vi "look up indices.vi"(8 "error in":errorcluster, 9 "output dictionary":refnum<class "data dictionary.lvclass">, 10 "input dictionary":refnum<class "data dictionary.lvclass">, 11 "slave data subsets":T4[](array[typedef])) -> (0 "error out":errorcluster, 2 "outputs":T1[](array[typedef]), 3 "inputs":T1[](array[typedef]))   [LabVIEW 2013, in "Profibus Module runtime.lvclass"]
uses:
  Profibus Module runtime.lvclass
  <vilib>/NI/Tag Bus/dictionary/data dictionary.lvclass
  required data sets.ctl
  channel/Profibus channel.lvclass
  profibus slave configuration.ctl
  profibus mapping configuration.ctl
  <vilib>/NI/Tag Bus/tag/Data Type.ctl
  channel/Profibus channel.lvclass/Profibus channel.ctl
  <vilib>/NI/Tag Bus/tag/tag descriptor.lvclass/tag descriptor.ctl
  channel/Read byte.vi
  channel/Read bit.vi
  <vilib>/NI/Tag Bus/tag/read tag name.vi
  <vilib>/NI/Tag Bus/tag/read data type.vi
  <vilib>/NI/Tag Bus/tag/tag descriptor.lvclass
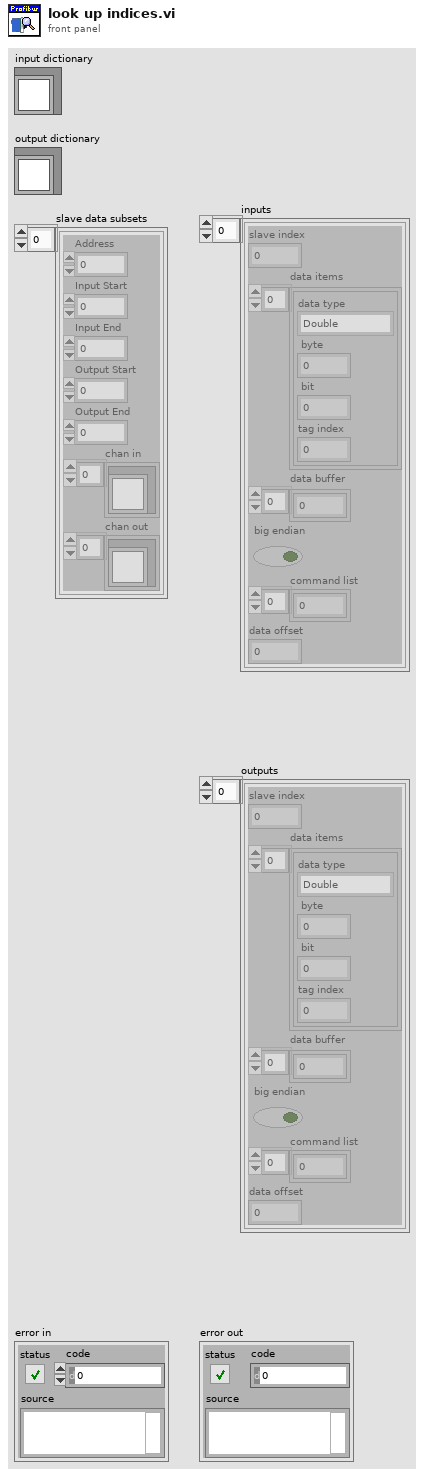
[diagram p1: front panel]
types:
  T1 = typedef "Profibus Module runtime.lvclass/profibus slave configuration.ctl" = cluster{"slave index":i8, "data items":T2[], "data buffer":u8[], "big endian":bool, "command list":u32[], "data offset":u8}
  T2 = typedef "Profibus Module runtime.lvclass/profibus mapping configuration.ctl" = cluster{"data type":T3, " byte":i32, " bit":i32, "tag index":i32}
  T3 = typedef "tag bus.lvlib/tag descriptor.lvclass/Data Type.ctl" = enum16{"Double", "Single", "I64", "I32", "I16", "I8", "U64", "U32", "U16", "U8", "Boolean", "String", "Array of Double", "Array of Single", "Array of I64", "Array of I32", "Array of I16", "Array of I8", "Array of U64", "Array of U32", "Array of U16", "Array of U8", "Array of Boolean", "Array of String"}
  T4 = typedef "Profibus Module runtime.lvclass/required data sets.ctl" = cluster{"Address":i8, "Input Start":u8, "Input End":u8, "Output Start":u8, "Output End":u8, "chan in":refnum<class "Profibus channel.lvclass">[], "chan out":refnum<class "Profibus channel.lvclass">[]}
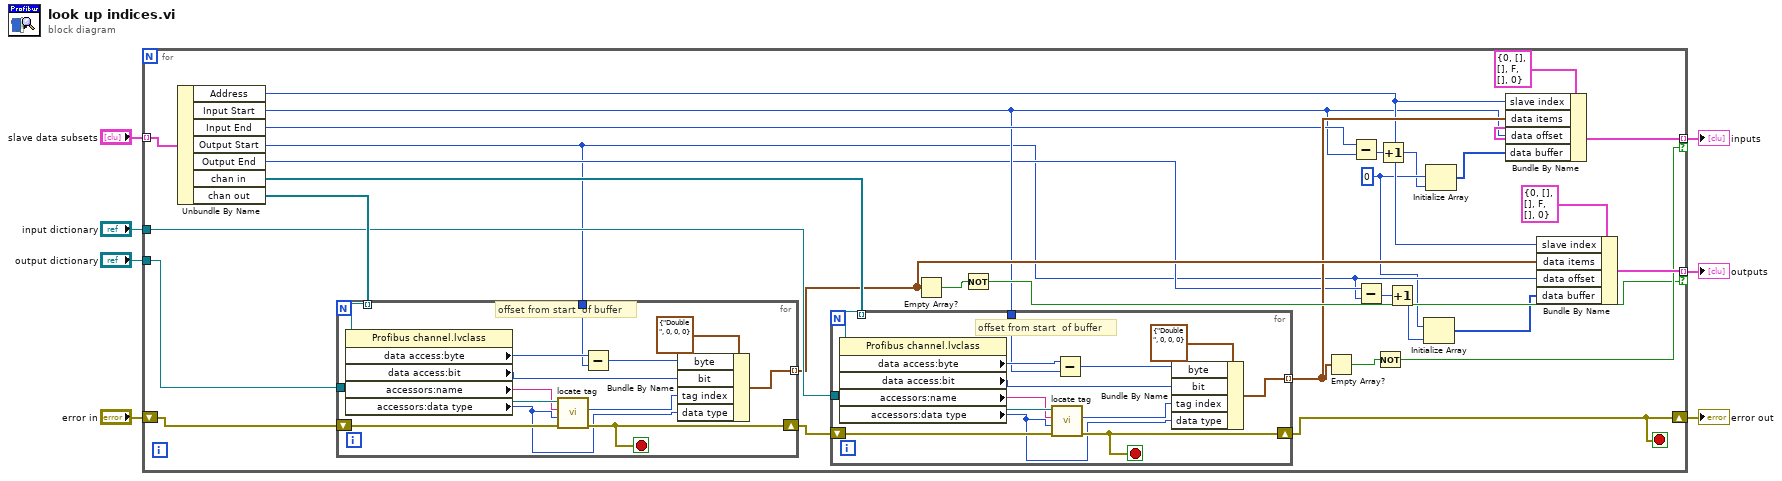
[diagram p0: block diagram]
diagram:
  n1 = for {
    tunnel: "slave data subsets" -> [w37] mode=indexing
    shift-right: [w22] -> w5
    shift-left: "error in" -> [w36]
    tunnel: "input dictionary" -> [w32]
    tunnel: "output dictionary" -> [w34]
    tunnel: [w26] -> w2 mode=indexing if=w24
    tunnel: [w25] -> w1 mode=indexing if=w23
    stop <- w22 stop-if-true
    w12 = u8 0
    n2 = Unbundle By Name(w37) -> ("Address"=w19:i8, "Input Start"=w17:u8, "Input End"=w18:u8, "Output Start"=w15:u8, "Output End"=w16:u8, "chan in"=w31:refnum<class "Profibus channel.lvclass">[], "chan out"=w35:refnum<class "Profibus channel.lvclass">[])
    n3 = for {
      tunnel: w35 -> [w63] mode=indexing
      tunnel: w34 -> [w61]
      shift-right: [w59] -> w33
      shift-left: w36 -> [w62]
      tunnel: [w57] -> w21 mode=indexing
      tunnel: w15 -> [w51]
      stop <- w59 stop-if-true
      # "offset from start  of buffer"
      n4 = property class="Profibus channel.lvclass"(reference=w63) -> ("data access:byte"=w53:i32, "data access:bit"=w54:i32, "accessors:name"=w60:string, "accessors:data type"=w55:T3)  [unwired: 1 in, 2 out]
      n5 = call <vilib>:"locate tag.vi"("error in"=w62, "data type"=w55, "name"=w60, "data dictionary in"=w61) -> ("error out"=w59:errorcluster, "index"=w56:i32)  [unwired: 5 in, 1 out]
      n6 = Subtract(x=w53, y=w51) -> (x-y=w52:i32)
      n7 = Bundle By Name(cluster=T2 {"data type"=enum."Double", " byte"=0, " bit"=0, "tag index"=0} ("data items"), "byte"=w52, "bit"=w54, "tag index"=w56, "data type"=w55) -> (w57:T2)
    }
    n8 = for {
      tunnel: w31 -> [w50] mode=indexing
      tunnel: w32 -> [w48]
      shift-right: [w46] -> w22
      shift-left: w33 -> [w49]
      tunnel: [w44] -> w20 mode=indexing
      tunnel: w17 -> [w38]
      stop <- w46 stop-if-true
      # "offset from start  of buffer"
      n9 = property class="Profibus channel.lvclass"(reference=w50) -> ("data access:byte"=w40:i32, "data access:bit"=w41:i32, "accessors:name"=w47:string, "accessors:data type"=w42:T3)  [unwired: 1 in, 2 out]
      n10 = call <vilib>:"locate tag.vi"("error in"=w49, "data type"=w42, "name"=w47, "data dictionary in"=w48) -> ("error out"=w46:errorcluster, "index"=w43:i32)  [unwired: 5 in, 1 out]
      n11 = Subtract(x=w40, y=w38) -> (x-y=w39:i32)
      n12 = Bundle By Name(cluster=T2 {"data type"=enum."Double", " byte"=0, " bit"=0, "tag index"=0} ("data items"), "byte"=w39, "bit"=w41, "tag index"=w43, "data type"=w42) -> (w44:T2)
    }
    n13 = Empty Array?(array=w21) -> (empty?=w27:bool)
    n14 = Not(x=w27) -> (.not. x?=w23:bool)
    n15 = Empty Array?(array=w20) -> (empty?=w28:bool)
    n16 = Subtract(x=w18, y=w17) -> (x-y=w13:u8)
    n17 = Subtract(x=w16, y=w15) -> (x-y=w10:u8)
    n18 = Not(x=w28) -> (.not. x?=w24:bool)
    n19 = Increment(x=w13) -> (x+1=w9:u8)
    n20 = Increment(x=w10) -> (x+1=w8:u8)
    n21 = Initialize Array(w12, w8) -> (w11:u8[])
    n22 = Initialize Array(w12, w9) -> (w14:u8[])
    n23 = Bundle By Name(cluster=T1 {"slave index"=0, "data items"=[], "data buffer"=[], "big endian"=FALSE, "command list"=[], "data offset"=0} ("slave configuration"), "slave index"=w19, "data items"=w20, "data offset"=w17, "data buffer"=w14) -> (w26:T1)
    n24 = Bundle By Name(cluster=T1 {"slave index"=0, "data items"=[], "data buffer"=[], "big endian"=FALSE, "command list"=[], "data offset"=0} ("slave configuration"), "slave index"=w19, "data items"=w21, "data offset"=w15, "data buffer"=w11) -> (w25:T1)
  }
  "error out" <- w5
  "outputs" <- w1
  "inputs" <- w2
